vi "Convert SN data to SN bytes.vi"(11 "SN":u32) -> (3 "SN Data Bytes":u8[](array[numeric]) format="%.0x")   [LabVIEW 2023]
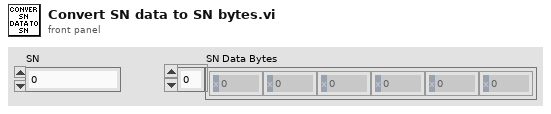
[diagram p1: front panel]
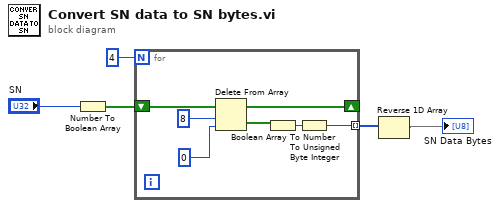
[diagram p0: block diagram]
diagram:
  n1 = Number To Boolean Array(number="SN") -> (Boolean array=w4:bool[])
  n2 = for {
    N: 4 -> [_]
    shift-right: [w12] -> _
    shift-left: w4 -> [w11]
    tunnel: [w6] -> w2 mode=indexing
    n3 = Delete From Array(array=w11, length=8, index=0) -> (deleted portion=w8:bool[], array with subset deleted=w12:bool[])
    n4 = Boolean Array To Number(Boolean array=w8) -> (number=w7:u32)
    n5 = To Unsigned Byte Integer(number=w7) -> (unsigned 8bit integer=w6:u8)
  }
  n6 = Reverse 1D Array(array=w2) -> (reversed array=→"SN Data Bytes":u8[])
